vi "nCr using while loop.vi"() -> ()   [LabVIEW 2024]
panel:
  in  "r":i32
  out "nCr":i32
  out "nPr":i32
  in  "n":i32
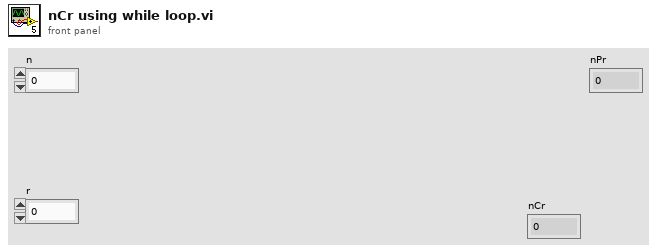
[diagram p1: front panel]
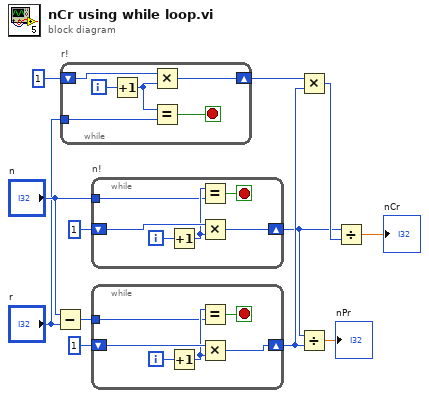
[diagram p0: block diagram]
diagram:
  n1 = Subtract(x="n", y="r") -> (x-y=w8:i32)
  n2 = while "r!" {
    shift-right: [w16] -> w1
    shift-left: 1 -> [w17]
    tunnel: "r" -> [w13]
    i -> [w18]
    stop <- w14 stop-if-true
    n3 = Increment(x=w18) -> (x+1=w15:i32)
    n4 = Multiply(x=w17, y=w15) -> (x*y=w16:i32)
    n5 = Equal?(x=w15, y=w13) -> (x = y?=w14:bool)
  }
  n6 = while "n!" {
    shift-right: [w22] -> w3
    shift-left: 1 -> [w23]
    tunnel: "n" -> [w19]
    i -> [w24]
    stop <- w20 stop-if-true
    n7 = Increment(x=w24) -> (x+1=w21:i32)
    n8 = Equal?(x=w21, y=w19) -> (x = y?=w20:bool)
    n9 = Multiply(x=w23, y=w21) -> (x*y=w22:i32)
  }
  n10 = while {
    shift-right: [w28] -> w5
    shift-left: 1 -> [w29]
    tunnel: w8 -> [w25]
    i -> [w30]
    stop <- w26 stop-if-true
    n11 = Increment(x=w30) -> (x+1=w27:i32)
    n12 = Equal?(x=w27, y=w25) -> (x = y?=w26:bool)
    n13 = Multiply(x=w29, y=w27) -> (x*y=w28:i32)
  }
  n14 = Multiply(x=w1, y=w5) -> (x*y=w4:i32)
  n15 = Divide(x=w3, y=w5) -> (x/y=→"nPr":dbl)
  n16 = Divide(x=w3, y=w4) -> (x/y=→"nCr":dbl)
